vi "GetLowPrioritySensors.vi"   [LabVIEW 2019]
doc: "All low priority sensor reads should be placed in this VI."
uses:
  refnums.vi
  GRNF_AI.vi
  GRNF_Compressor.vi
  sensors.vi
  GRNF_GenericMotor.vi
  robotprofile.vi
  GRNF_CTREMotor.vi
  <vilib>/Rock Robotics/WPI/ThirdParty/Phoenix-LabVIEW/Motor Controller/Get/CTRE_Phoenix_MotorController_GetTemperature.vi
types:
  T1 = typedef "WPI_MotorControlDeviceRef.ctl" = cluster{"DeviceStatus":errorcluster, "Type":T2, "PWM":cluster{"PWM Channel":T3, "DeadBand":T4}, "CAN":cluster{"Device Number":u8, "SetOutput VI Ref":variant, "GetOutput VI Ref":variant, "Enable VI Ref":variant, "Disable VI Ref":variant, "Data":variant}, "Invert":bool, "DIO PWM":cluster{"PWM \"Enable\" Channel":T3, "DIOChannel":T5, "PWM Rate":dbl}}
  T2 = typedef "WPI_MotorControlType.ctl" = enum16{"PWM", "CAN", "DIO PWM"}
  T3 = typedef "FPGA_DIOPWMChannel.ctl" = enum8{"PWM 0", "PWM 1", "PWM 2", "PWM 3", "PWM 4", "PWM 5", "PWM 6", "PWM 7", "PWM 8", "PWM 9", "PWM MXP 0", "PWM MXP 1", "PWM MXP 2", "PWM MXP 3", "PWM MXP 4", "PWM MXP 5", "PWM MXP 6", "PWM MXP 7", "PWM MXP 8", "PWM MXP 9", "Invalid"}
  T4 = typedef "WPI_PWMDeadband.ctl" = cluster{"Name":string, "maxPositivePwm":i32, "minPositivePwm":i32, "centerPwm":i32, "maxNegativePwm":i32, "minNegativePwm":i32, "angularRange":u16}
  T5 = typedef "FPGA_DIOChannel.ctl" = enum8{"DIO 0", "DIO 1", "DIO 2", "DIO 3", "DIO 4", "DIO 5", "DIO 6", "DIO 7", "DIO 8", "DIO 9", "DIO MXP 0", "DIO MXP 1", "DIO MXP 2", "DIO MXP 3", "DIO MXP 4", "DIO MXP 5", "DIO MXP 6", "DIO MXP 7", "DIO MXP 8", "DIO MXP 9", "DIO MXP 10", "DIO MXP 11", "DIO MXP 12", "DIO MXP 13", "DIO MXP 14", "DIO MXP 15", "SPI Port CS1", "SPI Port CS2", "SPI Port CS3", "SPI Port MISO", "SPI Port MOSI", "Invalid"}
  T6 = typedef "WPI_CompressorDevRef.ctl" = cluster{"DevStatus":errorcluster, "Pneumatics Control Module":u8}
  T7 = typedef "WPI_AnalogChannelDevRef.ctl" = cluster{"DevStatus":errorcluster, "Analog Channel":T8}
  T8 = typedef "FPGA_AIChannel.ctl" = enum8{"AI 0", "AI 1", "AI 2", "AI 3", "AI MXP 0", "AI MXP 1", "AI MXP 2", "AI MXP 3", "Invalid"}
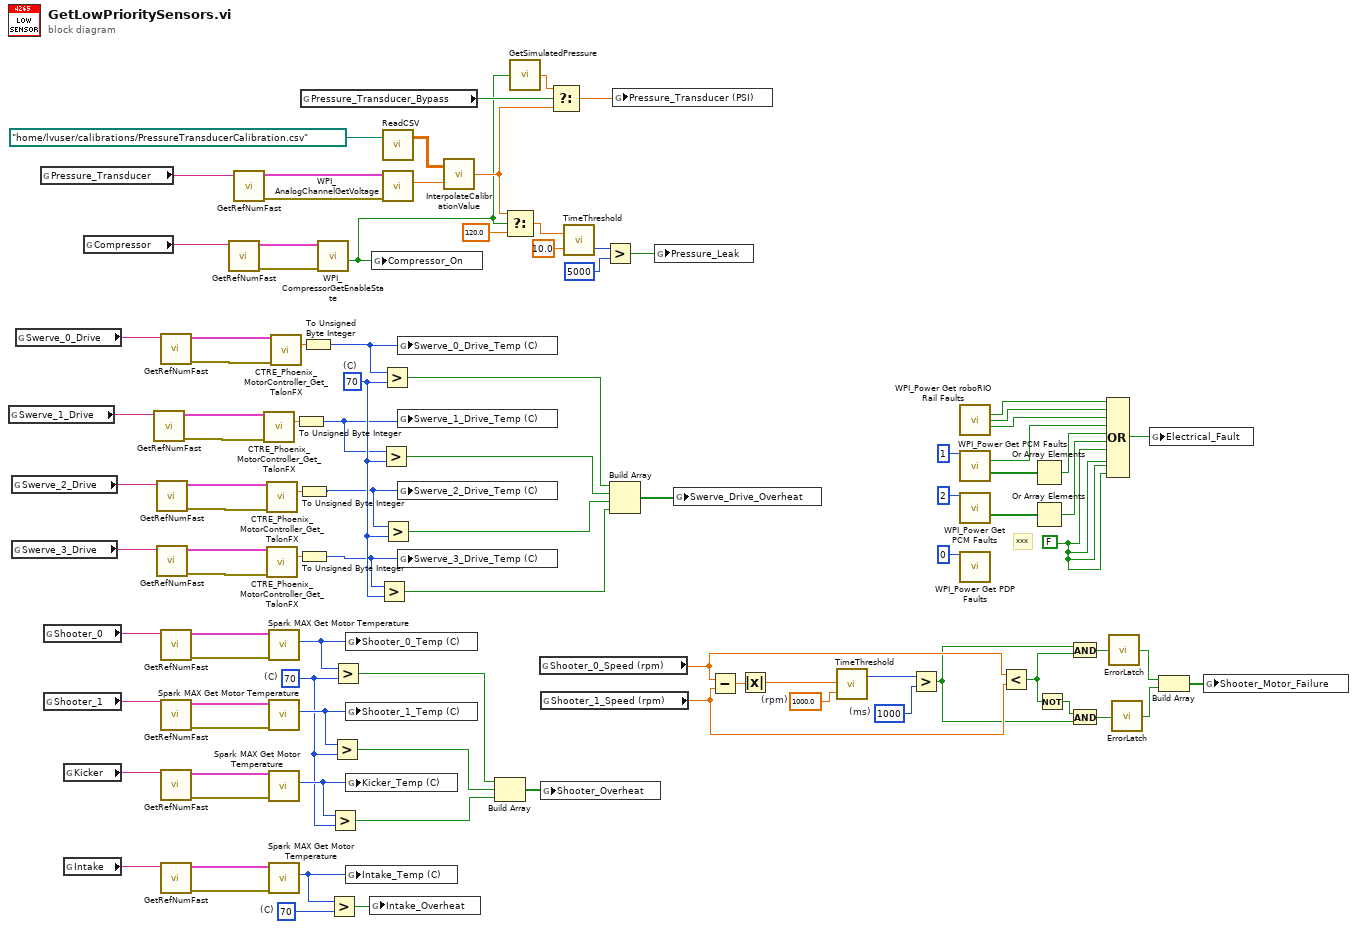
[diagram p0: block diagram]
diagram:
  w25 = FALSE
  w56 = u8 70  # (C)
  w71 = u32 1000  # (ms)
  w73 = 1000.0  # (rpm)
  w59 = u8 70  # (C)
  w86 = u8 70  # (C)
  # "***"
  n1 = global read "refnums.vi" "Swerve_1_Drive"() -> (w15:string)
  n2 = global read "refnums.vi" "Swerve_2_Drive"() -> (w11:string)
  n3 = global read "refnums.vi" "Swerve_3_Drive"() -> (w7:string)
  n4 = global read "refnums.vi" "Swerve_0_Drive"() -> (w50:string)
  n5 = global read "refnums.vi" "Pressure_Transducer"() -> (w51:string)
  n6 = global read "refnums.vi" "Shooter_0"() -> (w43:string)
  n7 = global read "refnums.vi" "Shooter_1"() -> (w42:string)
  n8 = global read "refnums.vi" "Kicker"() -> (w41:string)
  n9 = global read "refnums.vi" "Intake"() -> (w38:string)
  n10 = global read "refnums.vi" "Compressor"() -> (w88:string)
  n11 = call-poly "GetRefNumFast.vi"("RefNum Name"=w15) -> ("Error"=w13:errorcluster, "Device Reference"=w14:T1)  [unwired: 5 in]
  n12 = call-poly "GetRefNumFast.vi"("RefNum Name"=w11) -> ("Error"=w9:errorcluster, "Device Reference"=w10:T1)  [unwired: 5 in]
  n13 = call-poly "GetRefNumFast.vi"("RefNum Name"=w7) -> ("Error"=w5:errorcluster, "Device Reference"=w6:T1)  [unwired: 5 in]
  n14 = call-poly "GetRefNumFast.vi"("RefNum Name"=w50) -> ("Error"=w18:errorcluster, "Device Reference"=w19:T1)  [unwired: 5 in]
  n15 = call-poly "GetRefNumFast.vi"("RefNum Name"=w43) -> ("Error"=w48:errorcluster, "Device Reference"=w49:T1)  [unwired: 5 in]
  n16 = call-poly "GetRefNumFast.vi"("RefNum Name"=w42) -> ("Error"=w46:errorcluster, "Device Reference"=w47:T1)  [unwired: 5 in]
  n17 = call-poly "GetRefNumFast.vi"("RefNum Name"=w41) -> ("Error"=w44:errorcluster, "Device Reference"=w45:T1)  [unwired: 5 in]
  n18 = call-poly "GetRefNumFast.vi"("RefNum Name"=w38) -> ("Error"=w39:errorcluster, "Device Reference"=w40:T1)  [unwired: 5 in]
  n19 = call-poly "GetRefNumFast.vi"("RefNum Name"=w88) -> ("Error"=w54:errorcluster, "Device Reference"=w87:T6)  [unwired: 5 in]
  n20 = call-poly "GetRefNumFast.vi"("RefNum Name"=w51) -> ("Error"=w52:errorcluster, "Device Reference"=w53:T7)  [unwired: 5 in]
  n21 = call-poly <vilib>:"CTRE_Phoenix_MotorController_Get_TalonFX.vi"("PhoenixMotorControlDevRef"=w14, "error in"=w13) -> ("Temperature (C)"=w12:dbl)  [unwired: 11 in, 2 out]
  n22 = call-poly <vilib>:"CTRE_Phoenix_MotorController_Get_TalonFX.vi"("PhoenixMotorControlDevRef"=w10, "error in"=w9) -> ("Temperature (C)"=w8:dbl)  [unwired: 11 in, 2 out]
  n23 = call-poly <vilib>:"CTRE_Phoenix_MotorController_Get_TalonFX.vi"("PhoenixMotorControlDevRef"=w6, "error in"=w5) -> ("Temperature (C)"=w4:dbl)  [unwired: 11 in, 2 out]
  n24 = call <vilib>:"Spark MAX Get Motor Temperature.vi"("error in (no error)"=w48, "MotorControlDevRef in"=w49) -> ("Motor Temperature"=w80:u8)  [unwired: 6 in, 3 out]
  n25 = call <vilib>:"Spark MAX Get Motor Temperature.vi"("error in (no error)"=w46, "MotorControlDevRef in"=w47) -> ("Motor Temperature"=w79:u8)  [unwired: 6 in, 3 out]
  n26 = call <vilib>:"Spark MAX Get Motor Temperature.vi"("error in (no error)"=w44, "MotorControlDevRef in"=w45) -> ("Motor Temperature"=w60:u8)  [unwired: 6 in, 3 out]
  n27 = call <vilib>:"Spark MAX Get Motor Temperature.vi"("error in (no error)"=w39, "MotorControlDevRef in"=w40) -> ("Motor Temperature"=w57:u8)  [unwired: 6 in, 3 out]
  n28 = call-poly <vilib>:"CTRE_Phoenix_MotorController_Get_TalonFX.vi"("PhoenixMotorControlDevRef"=w19, "error in"=w18) -> ("Temperature (C)"=w17:dbl)  [unwired: 11 in, 2 out]
  n29 = To Unsigned Byte Integer(number=w12) -> (unsigned 8bit integer=w1:u8)
  n30 = To Unsigned Byte Integer(number=w8) -> (unsigned 8bit integer=w3:u8)
  n31 = To Unsigned Byte Integer(number=w4) -> (unsigned 8bit integer=w2:u8)
  n32 = global read "robotprofile.vi" "Pressure_Transducer_Bypass"() -> (w24:bool)
  n33 = To Unsigned Byte Integer(number=w17) -> (unsigned 8bit integer=w16:u8)
  n34 = call <vilib>:"WPI_CompressorGetEnableState.vi"("error in (no error)"=w54, "CompressorDevRef"=w87) -> ("Compressor Running"=w21:bool)  [unwired: 6 in, 3 out]
  n35 = Greater?(x=w57, y=w56) -> (0:w55:bool)
  n36 = Greater?(x=w60, y=w59) -> (0:w58:bool)
  n37 = Greater?(x=w79, y=w59) -> (0:w77:bool)
  n38 = Greater?(x=w80, y=w59) -> (0:w78:bool)
  n39 = global write "sensors.vi" "Shooter_0_Temp (C)"(w80) -> ()
  n40 = global write "sensors.vi" "Shooter_1_Temp (C)"(w79) -> ()
  n41 = global write "sensors.vi" "Kicker_Temp (C)"(w60) -> ()
  n42 = global write "sensors.vi" "Intake_Temp (C)"(w57) -> ()
  n43 = global write "sensors.vi" "Intake_Overheat"(w55) -> ()
  n44 = global write "sensors.vi" "Compressor_On"(w21) -> ()
  n45 = Greater?(x=w2, y=w86) -> (0:w82:bool)
  n46 = Greater?(x=w1, y=w86) -> (0:w84:bool)
  n47 = Greater?(x=w16, y=w86) -> (0:w85:bool)
  n48 = call "ReadCSV.vi"("File Path (.csv)"=path "/home/lvuser/calibrations/PressureTransducerCalibration.csv" ("path")) -> ("Data (index by row)"=w90:dbl[][])  [unwired: 1 in, 1 out]
  n49 = call <vilib>:"WPI_AnalogChannelGetVoltage.vi"("error in (no error)"=w52, "AIDeviceRef"=w53) -> ("Voltage"=w89:dbl)  [unwired: 7 in, 2 out]
  n50 = Greater?(x=w3, y=w86) -> (0:w83:bool)
  n51 = global write "sensors.vi" "Swerve_0_Drive_Temp (C)"(w16) -> ()
  n52 = global write "sensors.vi" "Swerve_1_Drive_Temp (C)"(w1) -> ()
  n53 = global write "sensors.vi" "Swerve_2_Drive_Temp (C)"(w3) -> ()
  n54 = global write "sensors.vi" "Swerve_3_Drive_Temp (C)"(w2) -> ()
  n55 = call "InterpolateCalibrationValue.vi"("Input"=w89, "Calibration Data"=w90) -> ("Interpolated Output"=w23:dbl)
  n56 = Build Array(w78, w77, w58) -> (w76:bool[])
  n57 = Select(t=w23, s=w21, f=120.0) -> (s? t:f=w94:dbl)
  n58 = call "GetSimulatedPressure.vi"("Compressor On"=w21) -> ("Simulated Pressure Transducer"=w20:dbl)
  n59 = global read "sensors.vi" "Shooter_0_Speed (rpm)"() -> (w70:dbl)
  n60 = global read "sensors.vi" "Shooter_1_Speed (rpm)"() -> (w69:dbl)
  n61 = global write "sensors.vi" "Shooter_Overheat"(w76) -> ()
  n62 = Select(t=w20, s=w24, f=w23) -> (s? t:f=w22:dbl)
  n63 = call "TimeThreshold.vi"("Threshold"=10.0, "Current Value"=w94) -> ("Time Below Threshold (ms)"=w93:u32)  [unwired: 1 out]
  n64 = Greater?(x=w93, y=u32 5000) -> (0:w91:bool)
  n65 = Build Array(w85, w84, w83, w82) -> (w81:bool[])
  n66 = global write "sensors.vi" "Pressure_Transducer (PSI)"(w22) -> ()
  n67 = global write "sensors.vi" "Pressure_Leak"(w91) -> ()
  n68 = global write "sensors.vi" "Swerve_Drive_Overheat"(w81) -> ()
  n69 = Subtract(x=w70, y=w69) -> (x-y=w75:dbl)
  n70 = Absolute Value(x=w75) -> (abs(x)=w74:dbl)
  n71 = call "TimeThreshold.vi"("Threshold"=w73, "Current Value"=w74) -> ("Time Above Threshold (ms)"=w72:u32)  [unwired: 1 out]
  n72 = Greater?(x=w72, y=w71) -> (0:w67:bool)
  n73 = call <vilib>:"WPI_Power Get roboRIO Rail Faults.vi"() -> ("3.3V User Rail Short"=w37:bool, "5 V User Rail Short"=w36:bool, "6 V User Rail Short"=w35:bool)  [unwired: 10 in, 3 out]
  n74 = call <vilib>:"WPI_Power Get PCM Faults.vi"("Pneumatics Control Module (0)"=u8 1) -> ("Compressor Fault"=w34:bool, "All Solenoid Faults"=w32:bool[])  [unwired: 11 in, 2 out]
  n75 = call <vilib>:"WPI_Power Get PCM Faults.vi"("Pneumatics Control Module (0)"=u8 2) -> ("All Solenoid Faults"=w30:bool[])  [unwired: 11 in, 3 out]
  n76 = call <vilib>:"WPI_Power Get PDP Faults.vi"("Power Distribution Panel (0)"=u8 0) -> ()  [unwired: 10 in, 5 out]
  n77 = Less?(x=w70, y=w69) -> (x < y?=w66:bool)
  n78 = Or Array Elements(Boolean array=w32) -> (logical OR=w31:bool)
  n79 = Or Array Elements(Boolean array=w30) -> (logical OR=w28:bool)
  n80 = Not(x=w66) -> (.not. x?=w68:bool)
  n81 = And(x=w67, y=w66) -> (x .and. y?=w65:bool)
  n82 = And(x=w68, y=w67) -> (x .and. y?=w64:bool)
  n83 = Compound Arithmetic op=OR(w37, w36, w35, w34, w31, w28, w25, w25, w25, w25) -> (w27:bool)
  n84 = call "ErrorLatch.vi"("Trigger"=w65) -> ("Latched"=w62:bool)
  n85 = call "ErrorLatch.vi"("Trigger"=w64) -> ("Latched"=w61:bool)
  n86 = global write "sensors.vi" "Electrical_Fault"(w27) -> ()
  n87 = Build Array(w62, w61) -> (w63:bool[])
  n88 = global write "sensors.vi" "Shooter_Motor_Failure"(w63) -> ()
